vi "SetDescription.vi"(6 "Label":string="Custom" caption="Label (\"Custom\")", 9 "Error in":errorcluster, 10 "Description":string) -> (1 "Error out":errorcluster)   [LabVIEW 2017, in "GPError.lvlib"]
doc: "Adds <B>Description</B> to an existing error or warning on <B>Error in</B>.\n\nIf <B>Error in</B> contains appended errors <B>Description</B> is only added to the primary error or warning.\n\nThis VI can be used to add details regarding the specific error (\"The file name was not found\", \"The operation exceeded the timeout value\", \"The result 4.68 was unexpected\" etc.). The optional <B>Label</B> lets you format the description for conformity with built-in LabVIEW error and warning messages like this: \"<Label>:\\s\\s<Description>\".\n\nThis VI is inlined, and it doesn't set any description if there is no error nor warning on <B>Error in</B>.\n\nSteen Schmidt\nGPower\n18/7 2013"
uses:
  GPError.lvlib
panel:
  # "Copyright © 2013\nSteen Schmidt, GPower\nSee enclosed license file for terms and conditions"
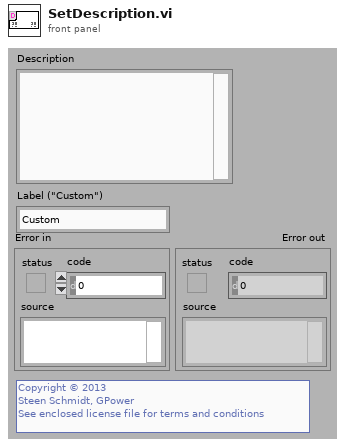
[diagram p1: front panel]
types:
  T1 = typedef "GPError.lvlib/ErrorType.ctl" = enum16{"No Error", "Error", "Warning", "Appended errors", "Appended warnings", "Appended mixed"}
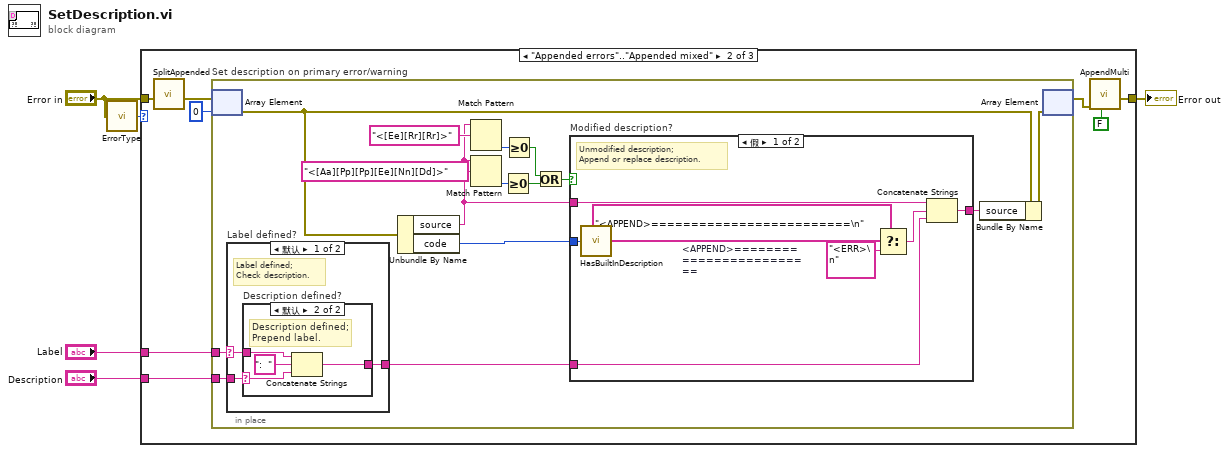
[diagram p0: block diagram]
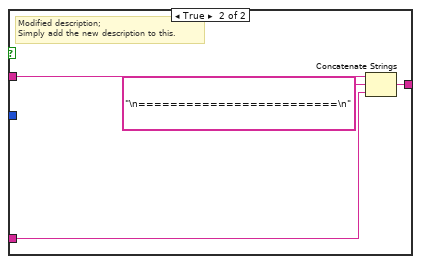
[diagram p5: hidden frame]
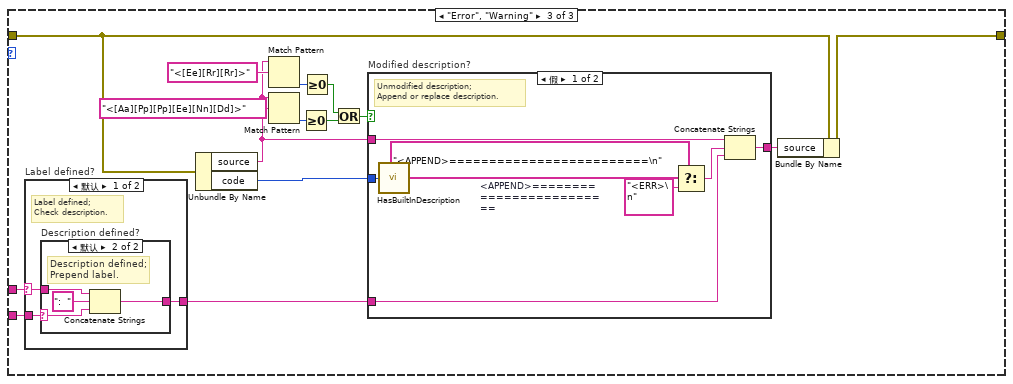
[diagram p6: hidden frame]
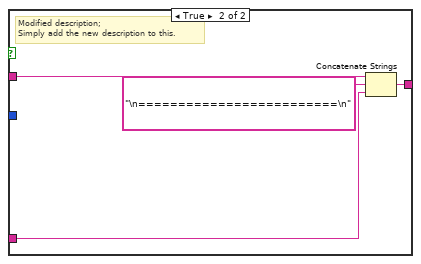
[diagram p9: hidden frame]
diagram:
  n1 = call "ErrorType.vi"("Error in"="Error in") -> ("Error type"=w1:T1)  [unwired: 4 in]
  n2 = case shown="\"Appended errors\"..\"Appended mixed\"" w1 {
    tunnel: [w6 w8 w51] -> w5
    tunnel: "Description" -> [_ w14 w53]
    tunnel: "Label" -> [_ w13 w52]
    tunnel: "Error in" -> [w6 w12 w50]
    frame "No Error" {
    }
    frame "Appended errors".."Appended mixed" {
      n3 = call "SplitAppended.vi"("Appended errors in"=w12) -> ("Errors out"=w11:errorcluster[])  [unwired: 10 in]
      n4 = in-place "Set description on primary error/warning" {
        in-place-border: w14 -> [w18]
        in-place-border: w13 -> [w17]
        n5 = in-place-array #1(w11, 0) -> (w16:errorcluster)
        n6 = case "Label defined?" shown="默认" w17 {
          selector: w17 -> [w32 _]
          tunnel: w18 -> [w30 w37]
          tunnel: [w31 w37] -> w19
          frame Default {
            # "Label defined;\nCheck description."
            n7 = case "Description defined?" shown="默认" w30 {
              selector: w30 -> [_ w33]
              tunnel: w32 -> [_ w36]
              tunnel: [_ w34] -> w31
              frame "" {
                # "No description defined;\nOmit label as well."
              }
              frame Default {
                # "Description defined;\nPrepend label."
                n8 = Concatenate Strings(w36, ":  ", w33) -> (w34:string)
              }
            }
          }
          frame "" {
            # "No label defined;\nJust use description."
          }
        }
        n9 = Unbundle By Name(w16) -> ("source"=w20:string, "code"=w22:i32)
        n10 = Match Pattern(string=w20, regular expression="<[Ee][Rr][Rr]>") -> (offset past match=w28:i32)  [unwired: 1 in, 3 out]
        n11 = Match Pattern(string=w20, regular expression="<[Aa][Pp][Pp][Ee][Nn][Dd]>") -> (offset past match=w26:i32)  [unwired: 1 in, 3 out]
        n12 = Greater Or Equal To 0?(x=w26) -> (x >= 0?=w24:bool)
        n13 = Greater Or Equal To 0?(x=w28) -> (x >= 0?=w25:bool)
        n14 = Or(x=w25, y=w24) -> (x .or. y?=w23:bool)
        n15 = case "Modified description?" shown="假" w23 {
          tunnel: w20 -> [w41 w49]
          tunnel: w19 -> [w39 w47]
          tunnel: w22 -> [w45 _]
          tunnel: [w38 w46] -> w21
          frame False {
            w43 = "<APPEND>=========================\n"  # <APPEND>=========================
            # "Unmodified description;\nAppend or replace description."
            n16 = call "HasBuiltInDescription.vi"("Error/warning code"=w45) -> ("Has built-in description?"=w44:bool)  [unwired: 4 in]
            n17 = Select(t=w43, s=w44, f="<ERR>\n") -> (s? t:f=w40:string)
            n18 = Concatenate Strings(w41, w40, w39) -> (w38:string)
          }
          frame True {
            # "Modified description;\nSimply add the new description to this."
            n19 = Concatenate Strings(w49, "\n=========================\n", w47) -> (w46:string)
          }
        }
        n20 = Bundle By Name(cluster=w16, "source"=w21) -> (w15:errorcluster)
        n21 = in-place-array #1(w15) -> (w9:errorcluster[])  [unwired: 1 out]
      }
      n22 = call "AppendMulti.vi"("Only append if new?"=FALSE, "Errors to append"=w9) -> ("Appended errors out"=w8:errorcluster)  [unwired: 9 in]
    }
    frame "Error", "Warning" {
      n23 = case "Label defined?" shown="默认" w52 {
        selector: w52 -> [w67 _]
        tunnel: w53 -> [w65 w72]
        tunnel: [w66 w72] -> w54
        frame Default {
          # "Label defined;\nCheck description."
          n24 = case "Description defined?" shown="默认" w65 {
            selector: w65 -> [_ w68]
            tunnel: w67 -> [_ w71]
            tunnel: [_ w69] -> w66
            frame "" {
              # "No description defined;\nOmit label as well."
            }
            frame Default {
              # "Description defined;\nPrepend label."
              n25 = Concatenate Strings(w71, ":  ", w68) -> (w69:string)
            }
          }
        }
        frame "" {
          # "No label defined;\nJust use description."
        }
      }
      n26 = Unbundle By Name(w50) -> ("source"=w55:string, "code"=w57:i32)
      n27 = Match Pattern(string=w55, regular expression="<[Ee][Rr][Rr]>") -> (offset past match=w63:i32)  [unwired: 1 in, 3 out]
      n28 = Match Pattern(string=w55, regular expression="<[Aa][Pp][Pp][Ee][Nn][Dd]>") -> (offset past match=w61:i32)  [unwired: 1 in, 3 out]
      n29 = Greater Or Equal To 0?(x=w61) -> (x >= 0?=w59:bool)
      n30 = Greater Or Equal To 0?(x=w63) -> (x >= 0?=w60:bool)
      n31 = Or(x=w60, y=w59) -> (x .or. y?=w58:bool)
      n32 = case "Modified description?" shown="假" w58 {
        tunnel: w55 -> [w76 w84]
        tunnel: w54 -> [w74 w82]
        tunnel: w57 -> [w80 _]
        tunnel: [w73 w81] -> w56
        frame False {
          w78 = "<APPEND>=========================\n"  # <APPEND>=========================
          # "Unmodified description;\nAppend or replace description."
          n33 = call "HasBuiltInDescription.vi"("Error/warning code"=w80) -> ("Has built-in description?"=w79:bool)  [unwired: 4 in]
          n34 = Select(t=w78, s=w79, f="<ERR>\n") -> (s? t:f=w75:string)
          n35 = Concatenate Strings(w76, w75, w74) -> (w73:string)
        }
        frame True {
          # "Modified description;\nSimply add the new description to this."
          n36 = Concatenate Strings(w84, "\n=========================\n", w82) -> (w81:string)
        }
      }
      n37 = Bundle By Name(cluster=w50, "source"=w56) -> (w51:errorcluster)
    }
  }
  "Error out" <- w5
